vi "file list from temperatures file V5.vi"(0 "sweep folder path  IN":path=path "/snowfall/Users/arcadi/Desktop/Ultrasound/Experiment/YBCO_4/Round1/Sweep12/June_2011/062511/221.16400K_300_3100_001_062511.dat", 1 "tfolder IN":T1={"tfolder path"=path "/snowfall/Users/arcadi/Desktop/Ultrasound/Experiment/YBCO_4/Round1/Sweep12/June_2011/062511/221.16400K_300_3100_001_062511.dat", "9folder path"=path "/snowfall/Users/arcadi/Desktop/Ultrasound/Experiment/YBCO_4/Round1/Sweep12/June_2011/062511/221.16400K_300_3100_001_062511.dat", "tfolder  -  file array"=[], "from index array"=[], "timestamp array"=[]}, 10 "action":T4(ring)=enum."update monotonic pieces", 11 "monotonic segments ON/OFF":bool=TRUE) -> (20 "sweep path array OUT":T3[](array[typedef]), 21 "tfolder OUT":T1={"tfolder path"=path "/snowfall/Users/arcadi/Desktop/Ultrasound/Experiment/YBCO_4/Round1/Sweep12/June_2011/062511/221.16400K_300_3100_001_062511.dat", "9folder path"=path "/snowfall/Users/arcadi/Desktop/Ultrasound/Experiment/YBCO_4/Round1/Sweep12/June_2011/062511/221.16400K_300_3100_001_062511.dat", "tfolder  -  file array"=[], "from index array"=[], "timestamp array"=[]}, 22 "OK":bool, 23 "temperature OUT":dbl[](array[numeric]), 24 "power  OUT":dbl[](array[numeric]), 25 "Magn Field  OUT":dbl[](array[numeric]), 26 "timestamp OUT":dbl[](array[numeric]))   [LabVIEW 2018]
uses:
  sweep file name.ctl
  tfolder.ctl
  tfolder -- monotonic segment.ctl
  array -- find monotonic segments -- testblock.vi
panel:
  out "last  mod OUT":timestamp[](array[timestamp])
  in  "file path OK":bool=TRUE
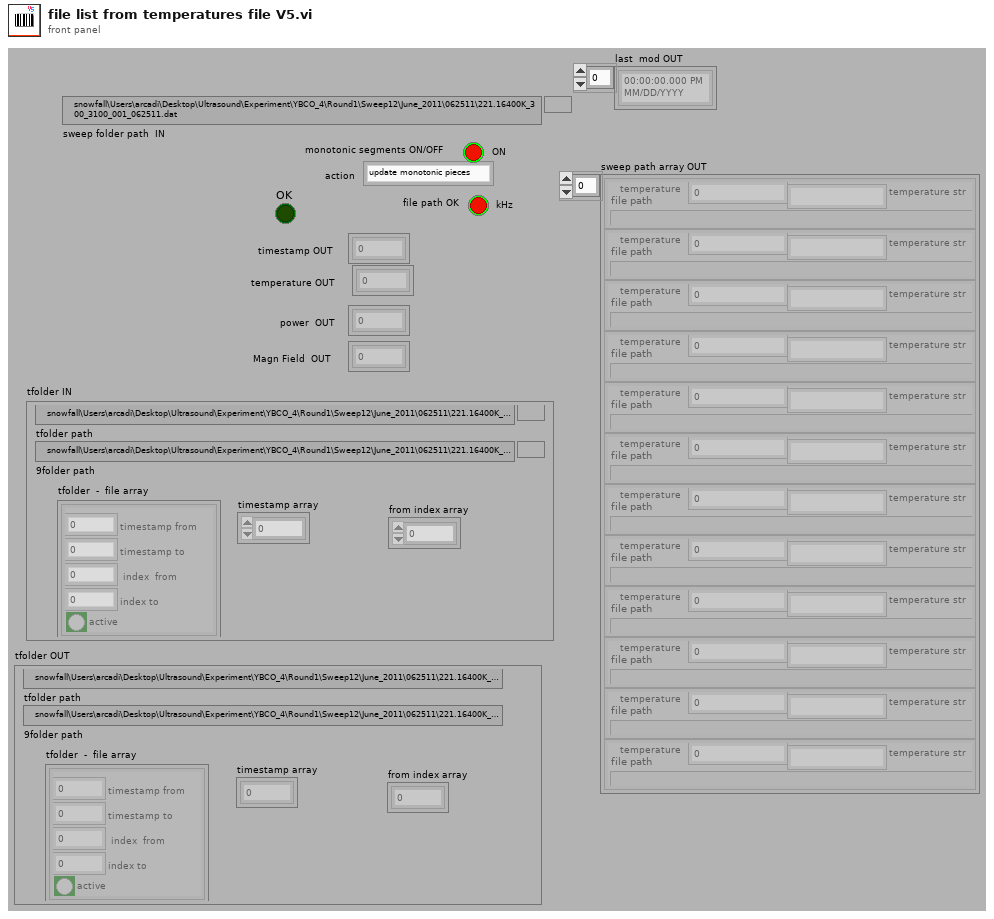
[diagram p1: front panel]
types:
  T1 = typedef "tfolder.ctl" = cluster{"tfolder path":path, "9folder path":path, "tfolder  -  file array":T2[], "from index array":i32[], "timestamp array":dbl[]}
  T2 = typedef "tfolder -- monotonic segment.ctl" = cluster{"timestamp from":dbl, "timestamp to":dbl, " index  from":i32, "index to":i32, "active":bool}
  T3 = typedef "sweep file name.ctl" = cluster{"temperature":dbl, "temperature str":string, "file path":path, "last mod":timestamp, "file name str":string, "mod time(min)":dbl, "file format":enum16{"", "ascii", "binary"}, "power(V)":dbl, "Magn Field(T) ":dbl}
  T4 = enum16{"new", "update range", "update monotonic pieces", "init", "check", "reset", ""}
  T5 = cluster{"index to":i32, "index from":i32, "up|dowm":enum16{"up", "down"}}
  T6 = typedef "array -- monotnic segment.ctl" = cluster{"to":i32, "from":i32, "up|dowm":enum16{"up", "down"}}
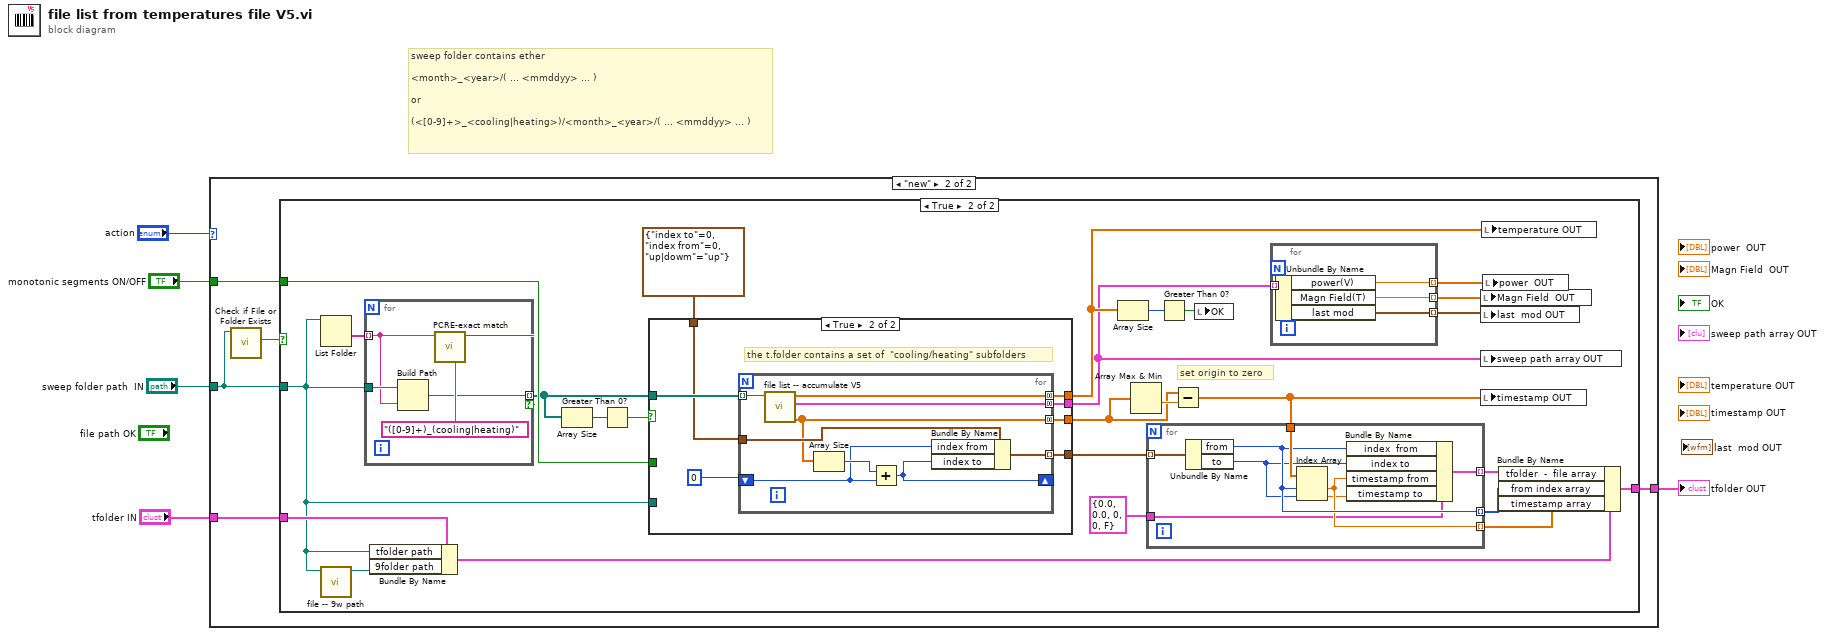
[diagram p0: block diagram]
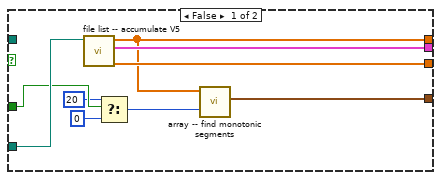
[diagram p4: hidden frame]
diagram:
  # "sweep folder contains ether \n\n<month>_<year>/( ... <mmddyy> ... ) \n\nor\n\n(<[0-9]+>_<cooling|heating>)/<month>_<year>/( ... <mmddyy> ... )"
  n1 = case shown="\"new\"" "action" {
    tunnel: "sweep folder path  IN" -> [_ w10]
    tunnel: "tfolder IN" -> [w6 w9]
    tunnel: [w6 w8] -> w2
    tunnel: "monotonic segments ON/OFF" -> [_ w7]
    frame "", Default {
    }
    frame "new" {
      n2 = call <vilib>:"Check if File or Folder Exists.vi"("path"=w10) -> ("file or folder exists?"=w11:bool)  [unwired: 8 in, 2 out]
      n3 = case shown="True" w11 {
        tunnel: w10 -> [_ w27]
        tunnel: w9 -> [w12 w35]
        tunnel: [w12 w33] -> w8
        tunnel: w7 -> [_ w31]
        frame False {
        }
        frame True {
          # "set origin to zero"
          n4 = List Folder(path=w27) -> (folder names=w38:string[])  [unwired: 3 in, 3 out]
          n5 = call "file -- 9w path.vi"("sweep folder"=w27) -> ("9w path"=w26:path)  [unwired: 10 in]
          n6 = for {
            tunnel: w38 -> [w78] mode=indexing
            tunnel: w27 -> [w79]
            tunnel: [w77] -> w25 mode=indexing if=w76
            n7 = Build Path(base path=w79, name or relative path=w78) -> (appended path=w77:path)
            n8 = call "PCRE-exact match.vi"("regular expression"="([0-9]+)_(cooling|heating)", "input string"=w78) -> ("exact match"=w76:bool)  [unwired: 7 in, 2 out]
          }
          n9 = Bundle By Name(cluster=w35, "tfolder path"=w27, "9folder path"=w26) -> (w19:T1)
          n10 = Array Size(array=w25) -> (size(s)=w37:i32)
          n11 = Greater Than 0?(x=w37) -> (x > 0?=w36:bool)
          n12 = case shown="True" w36 {
            tunnel: w25 -> [_ w66]
            tunnel: [w57 w64] -> w18
            tunnel: [w56 w61] -> w29
            tunnel: [w59 w62] -> w16
            tunnel: w27 -> [w58 _]
            tunnel: w31 -> [w55 _]
            tunnel: [w51 w65] -> w21
            tunnel: T5 {"index to"=0, "index from"=0, "up|dowm"=enum."up"} -> [_ w60]
            frame False {
              n13 = call "file list -- accumulate V5.vi"("tfolder path"=w58) -> ("timestamp"=w57:dbl[], "sweep file name array"=w59:T3[], "temperatures"=w56:dbl[])  [unwired: 8 in]
              n14 = Select(t=20, s=w55, f=0) -> (s? t:f=w54:i32)
              n15 = call "array -- find monotonic segments.vi"("min length of monotonic segment"=w54, "list of numbers"=w56) -> ("array of monotonic segments"=w51:T6[])  [unwired: 9 in]
            }
            frame True {
              # "the t.folder contains a set of  \"cooling/heating\" subfolders"
              n16 = for {
                tunnel: w66 -> [w75] mode=indexing
                shift-right: [w68] -> _
                shift-left: 0 ("dimension size") -> [w71]
                tunnel: w60 -> [w73]
                tunnel: [w72] -> w65 mode=indexing
                tunnel: [w67] -> w64 mode=concatenating
                tunnel: [w70] -> w62 mode=concatenating
                tunnel: [w69] -> w61 mode=concatenating
                n17 = call "file list -- accumulate V5.vi"("tfolder path"=w75) -> ("timestamp"=w67:dbl[], "sweep file name array"=w70:T3[], "temperatures"=w69:dbl[])  [unwired: 8 in]
                n18 = Array Size(array=w67) -> (size(s)=w74:i32)
                n19 = Add(x=w74, y=w71) -> (x+y=w68:i32)
                n20 = Bundle By Name(cluster=w73, "index from"=w71, "index to"=w68) -> (w72:T5)
              }
            }
          }
          n21 = Array Size(array=w29) -> (size(s)=w30:i32)
          n22 = Array Max & Min(array=w18) -> (min value=w34:dbl)  [unwired: 3 out]
          n23 = Greater Than 0?(x=w30) -> (x > 0?=w28:bool)
          n24 = Subtract(x=w18, y=w34) -> (x-y=w32:dbl[])
          n25 = for {
            tunnel: w21 -> [w50] mode=indexing
            tunnel: w32 -> [w49]
            tunnel: [w48] -> w24 mode=indexing
            tunnel: [w47] -> w23 mode=indexing
            tunnel: [w46] -> w22 mode=indexing
            tunnel: T2 {"timestamp from"=0.0, "timestamp to"=0.0, " index  from"=0, "index to"=0, "active"=FALSE} ("tfolder - monotonic segment") -> [w43]
            n26 = Unbundle By Name(w50) -> ("from"=w47:i32, "to"=w44:i32)
            n27 = Index Array(array=w49, index #1=w47, index #2=w44) -> (element #1=w46:dbl, element #2=w45:dbl)
            n28 = Bundle By Name(cluster=w43, "index  from"=w47, "index to"=w44, "timestamp from"=w46, "timestamp to"=w45) -> (w48:T2)
          }
          n29 = local write "OK"(w28) -> ()
          n30 = for {
            tunnel: w16 -> [w42] mode=indexing
            tunnel: [w41] -> w15 mode=indexing
            tunnel: [w40] -> w14 mode=indexing
            tunnel: [w39] -> w13 mode=indexing
            n31 = Unbundle By Name(w42) -> ("power(V)"=w41:dbl, "Magn Field(T)"=w39:dbl, "last mod"=w40:timestamp)
          }
          n32 = local write "Magn Field  OUT"(w13) -> ()
          n33 = local write "last  mod OUT"(w14) -> ()
          n34 = local write "sweep path array OUT"(w16) -> ()
          n35 = local write "timestamp OUT"(w32) -> ()
          n36 = local write "temperature OUT"(w29) -> ()
          n37 = local write "power  OUT"(w15) -> ()
          n38 = Bundle By Name(cluster=w19, "tfolder  -  file array"=w24, "from index array"=w23, "timestamp array"=w22) -> (w33:T1)
        }
      }
    }
  }
  "tfolder OUT" <- w2
